vi "guardadoarchivocompleto2.vi"(0 "nombre":string, 1 "lockin":dbl[](array[numeric]), 2 "multimetro":bool, 3 "CCD":dbl[][](array[numeric]), 5 "titulo grupo":string, 6 "voltaje":dbl[](array[numeric]), 7 "potenciometro":dbl[](array[numeric]), 8 "angulo":dbl[](array[numeric]), 9 "division":dbl[](array[numeric]), 10 "Enum":T1(ring), 11 "Orden":T2(array[ring])=[enum."espejos", enum."voltaje", enum."polarizador", enum."potenciometro "], 12 "polarizador":dbl[](array[numeric]), 13 "corriente":dbl[](array[numeric]), 14 "multim.":dbl[](array[numeric]), 15 "guardar corriente":bool) -> ()   [LabVIEW 2016]
doc: "En este subVI se realiza el guardado de la información de acuerdo con el dispositivo que se encuentre en penultimo lugar y si en ultimo lugar se encuentra la CCD. \n\nLas entradas son:\nLa cadena de nombre, en la que se especifica el nombre del archivo.\nLa cadena de nombre de los grupos que se van a realizar, en caso de que la cadena llegue vacía entoces no se forman ningún grupo."
uses:
  <vilib>/UPVI/lvhdf5/file.llb/LVH5F Operation.ctl
  <vilib>/Utility/miscctls.llb/LVRectTypeDef.ctl
  <vilib>/UPVI/lvhdf5/attribute.llb/LVH5A Operation.ctl
  <vilib>/UPVI/lvhdf5/group.llb/H5G_obj_t.ctl
  <vilib>/UPVI/lvhdf5/dataset.llb/LVH5D Operation.ctl
  <vilib>/UPVI/lvhdf5/identifier.llb/Not an HDF5 Refnum Constant.vi
  <vilib>/UPVI/lvhdf5/common.llb/To HDF5 Ref.vi
  <vilib>/UPVI/lvhdf5/group.llb/OpenCreateGroup (String).vi
  <vilib>/UPVI/lvhdf5/utility.llb/Select HDF5 Dialog.vi
  <vilib>/UPVI/lvhdf5/utility.llb/Select HDF5 Dialog (Object Only).vi
  <vilib>/UPVI/lvhdf5/dataset.llb/Simple H5Dwrite (Variant).vi
  <vilib>/UPVI/lvhdf5/attribute.llb/Write Multiple Attributes.vi
  <vilib>/UPVI/lvhdf5/dataset.llb/H5Dclose.vi
  <vilib>/UPVI/lvhdf5/dataset.llb/Write Dataset with Attributes.xnode
  <vilib>/UPVI/lvhdf5/library.llb/HDF5 Ref.ctl
  <vilib>/Utility/error.llb/Error Cluster From Error Code.vi
  <vilib>/UPVI/lvhdf5/dataset.llb/OpenCreateReplace Dataset by Element Type.vi
  <vilib>/UPVI/lvhdf5/dataspace.llb/H5Sselect_hyperslab.vi
  <vilib>/UPVI/lvhdf5/dataset.llb/H5Dwrite (Variant).vi
  <vilib>/UPVI/lvhdf5/dataset.llb/H5Dget_space.vi
  <vilib>/UPVI/lvhdf5/attribute.llb/private/LVH5AwriteWDTAttrs.vi
  <vilib>/UPVI/lvhdf5/dataspace.llb/H5Sclose.vi
  <vilib>/UPVI/lvhdf5/utility.llb/Select HDF5 Dialog (File and Object).vi
  <vilib>/Utility/VariantDataType/GetClusterInfo.vi
  <vilib>/Utility/VariantDataType/VariantType.lvlib
  <vilib>/Utility/VariantDataType/GetTypeInfo.vi
  <vilib>/UPVI/lvhdf5/attribute.llb/Cluster to Attribute Array.xnode
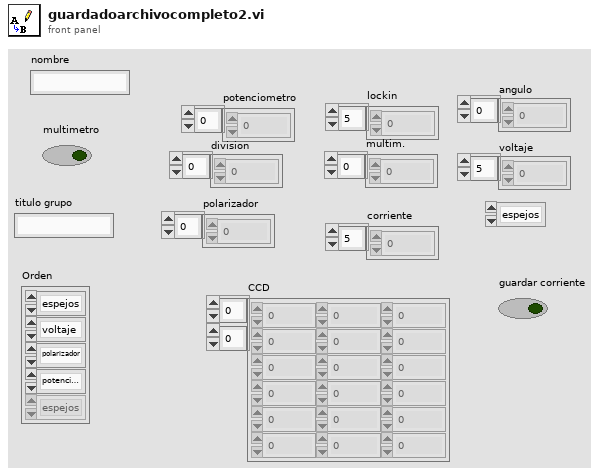
[diagram p1: front panel]
types:
  T1 = enum16{"espejos", "polarizador", "voltaje", "potenciometro ", "CCD", "lockin", "laser", "ninguno"}
  T2 = enum16{"espejos", "polarizador", "voltaje", "potenciometro ", "CCD", "lockin", "laser", "ninguno"}[]
  T3 = typedef "LVH5F Operation.ctl" = enum16{"open", "open or create", "create or replace", "create or replace (with confirmation)", "create", "open (read only)"}
  T4 = typedef "HDF5 Ref.ctl" = refnum<k1>
  T5 = typedef "LVH5A Operation.ctl" = enum16{"open", "replace", "create", "open or create", "create or replace", "create or replace with confirmation"}
  T6 = typedef "LVRectTypeDef.ctl" = cluster{"Left":i16, "Top":i16, "Right":i16, "Bottom":i16}
  T7 = cluster{"Behavior":enum32{"Invalid", "Default", "Floating", "Floating/Auto-Hide", "Modal"}, "Position":T6, "Center":bool, "Title":string}
  T8 = typedef "LVH5D Operation.ctl" = enum16{"open", "replace", "create", "open or create", "create or replace", "create or replace with confirmation"}
  T9 = typedef "H5G_obj_t.ctl" = i32
  T10 = cluster{"Object Types (any)":T9[], "Object Pattern":string}
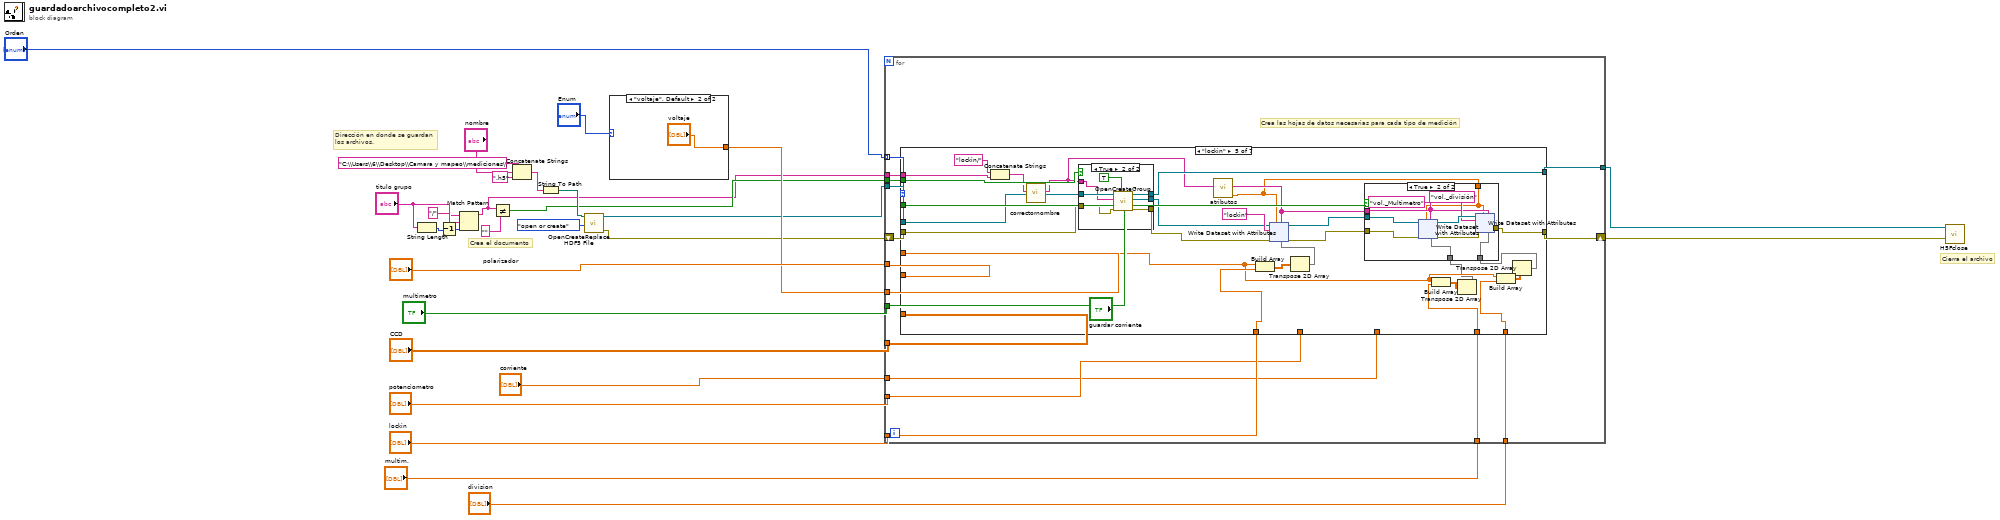
[diagram p0: block diagram]
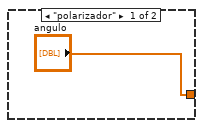
[diagram p2: hidden frame]
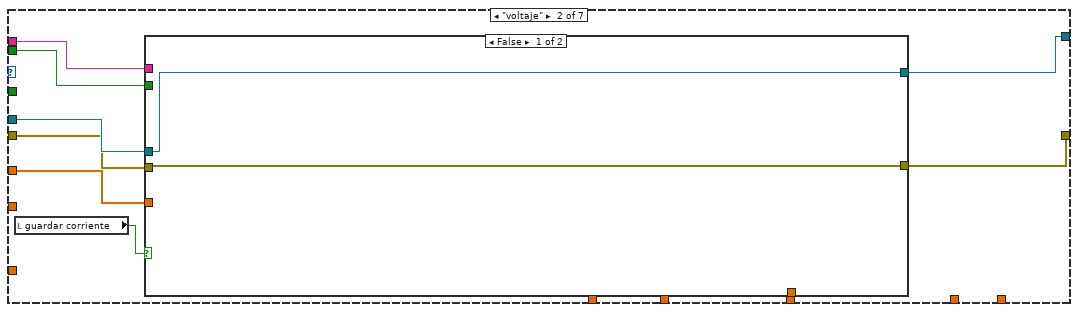
[diagram p4: hidden frame]
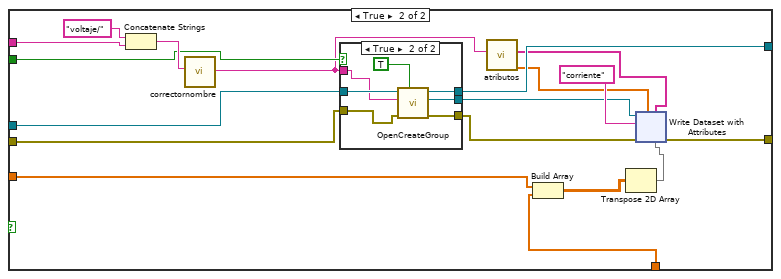
[diagram p5: hidden frame]
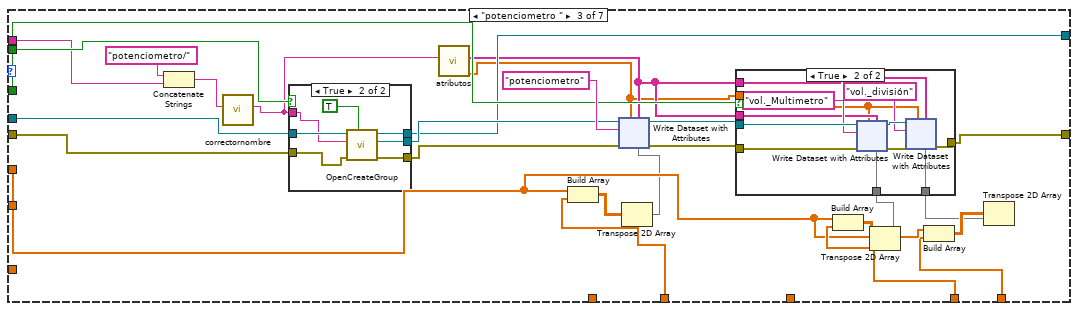
[diagram p7: hidden frame]
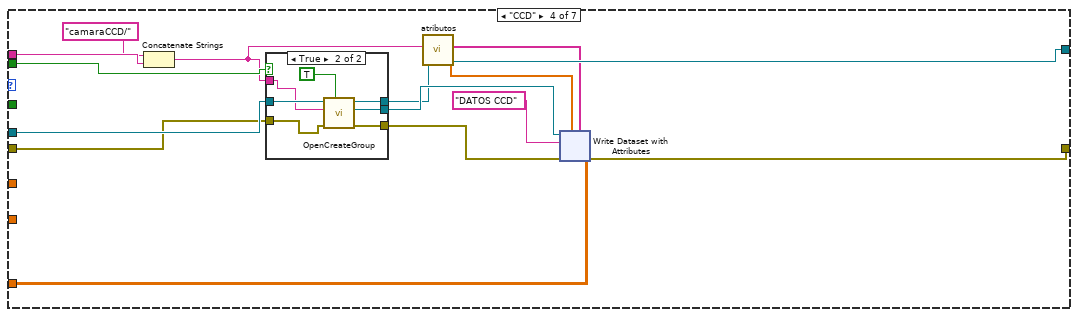
[diagram p10: hidden frame]
diagram:
  # "Dirección en donde se guardan \nlos archivos."
  # "Cierra el archivo"
  # "Crea el documento"
  n1 = String Length(string="titulo grupo") -> (length=w15:i32)
  n2 = Decrement(x=w15) -> (x-1=w16:i32)
  n3 = Match Pattern(string="titulo grupo", regular expression="/", offset (0)=w16) -> (before substring=w2:string)  [unwired: 3 out]
  n4 = Not Equal?(x=w2, y="") -> (x != y?=w3:bool)
  n5 = Concatenate Strings("C:\\Users\\6\\Desktop\\Camara y mapeo\\mediciones\\" ("string"), "nombre", ".h5" ("string")) -> (w24:string)
  n6 = String To Path(string=w24) -> (path=w23:path)
  n7 = call <vilib>:"OpenCreateReplace HDF5 File.vi"("function (open or create)"=LVH5F_Operation."open or create", "path"=w23) -> ("error out"=w4:errorcluster, "HDF5 Ref out"=w5:T4)  [unwired: 6 in]
  n8 = case shown="\"voltaje\", Default" "Enum" {
    tunnel: ["angulo" "voltaje"] -> w7
    frame "polarizador" {
    }
    frame "voltaje", Default {
    }
  }
  n9 = for {
    tunnel: "polarizador" -> [w45]
    tunnel: w5 -> [w44]
    tunnel: "Orden" -> [w43] mode=indexing
    tunnel: "lockin" -> [w41]
    tunnel: "potenciometro" -> [w40]
    tunnel: "corriente" -> [w39]
    tunnel: "multimetro" -> [w38]
    tunnel: "multim." -> [w37]
    tunnel: "CCD" -> [w36]
    shift-right: [w42] -> w21
    shift-left: w4 -> [w46]
    tunnel: "division" -> [w35]
    tunnel: w7 -> [w34]
    tunnel: w3 -> [w33]
    tunnel: w2 -> [w32]
    tunnel: [w31] -> w1
    # "Crea las hojas de datos necesarias para cada tipo de medición"
    n10 = case shown="\"lockin\"" w43 {
      tunnel: w46 -> [w48 w51 w393 w1319 w1645 w2560 w2562]
      tunnel: w45 -> [_ _ _ _ _ _ _]
      tunnel: w44 -> [w47 w52 w394 w1320 w1640 w2559 w2561]
      tunnel: [w48 w57 w404 w1325 w1652 w2560 w2562] -> w42
      tunnel: w41 -> [_ _ _ _ w1650 _ _]
      tunnel: w40 -> [_ _ w402 _ _ _ _]
      tunnel: w39 -> [_ w55 _ _ _ _ _]
      tunnel: w38 -> [_ _ w403 _ w1651 _ _]
      tunnel: w37 -> [_ _ w401 _ w1649 _ _]
      tunnel: w36 -> [_ _ _ w1323 _ _ _]
      tunnel: w35 -> [_ _ w399 _ w1648 _ _]
      tunnel: w34 -> [_ w56 w400 _ w1647 _ _]
      tunnel: w33 -> [_ w53 w397 w1315 w1642 _ _]
      tunnel: w32 -> [_ w54 w395 w1322 w1641 _ _]
      tunnel: [w47 w50 w390 w1316 w1639 w2559 w2561] -> w31
      frame "espejos", Default {
      }
      frame "voltaje" {
        n11 = local read "guardar corriente"() -> (w49:bool)
        n12 = case shown="False" w49 {
          tunnel: [w59 w76] -> w57
          tunnel: w56 -> [_ w75]
          tunnel: w55 -> [_ w74]
          tunnel: w54 -> [_ w71]
          tunnel: w53 -> [_ w70]
          tunnel: w52 -> [w58 w69]
          tunnel: w51 -> [w59 w68]
          tunnel: [w58 w65] -> w50
          frame False {
          }
          frame True {
            n13 = Concatenate Strings("voltaje/", w71) -> (w72:string)
            n14 = call "correctornombre.vi"("NUEVA"=w72) -> ("concatenated string"=w62:string)  [unwired: 10 in]
            n15 = case shown="True" w70 {
              tunnel: w69 -> [w373 w380]
              tunnel: w68 -> [w372 w379]
              tunnel: [w372 w378] -> w67
              tunnel: [w373 w377] -> w66
              tunnel: [w373 w375] -> w65
              tunnel: w62 -> [_ w374]
              frame False {
              }
              frame True {
                n16 = call-poly <vilib>:"OpenCreateGroup.vi"("Create if not found (F)"=TRUE, "error in (no error)"=w379, "Group"=w374, "HDF5 Ref"=w380) -> ("error out"=w378:errorcluster, "HDF5 Group Ref"=w377:T4, "HDF5 Ref out"=w375:T4)  [unwired: 5 in]
              }
            }
            n17 = call "atributos.vi"("titulo grupo"=w62) -> ("Array 2"=w60:dbl[], "Array"=w61:string[])  [unwired: 9 in]
            n18 = Build Array(w75, w74) -> (w63:dbl[][])
            n19 = Transpose 2D Array(2D array=w63) -> (transposed array=w64:dbl[][])
            n20 = xnode "Write Dataset with Attributes"("Dataset Path"="corriente", "error in (no error)"=w67, "HDF5 Path or Ref"=w66, "Attribute Name(s)"=w61, "Attribute Value(s)"=w60, "Data"=w64) -> ("error out"=w76:errorcluster)  [unwired: 2 in, 2 out]
          }
        }
      }
      frame "potenciometro " {
        n21 = Concatenate Strings("potenciometro/", w395) -> (w398:string)
        n22 = call "correctornombre.vi"("NUEVA"=w398) -> ("concatenated string"=w383:string)  [unwired: 10 in]
        n23 = case shown="True" w397 {
          tunnel: w394 -> [w703 w710]
          tunnel: w393 -> [w702 w709]
          tunnel: [w702 w708] -> w392
          tunnel: [w703 w707] -> w391
          tunnel: [w703 w705] -> w390
          tunnel: w383 -> [_ w704]
          frame False {
          }
          frame True {
            n24 = call-poly <vilib>:"OpenCreateGroup.vi"("Create if not found (F)"=TRUE, "error in (no error)"=w709, "Group"=w704, "HDF5 Ref"=w710) -> ("error out"=w708:errorcluster, "HDF5 Group Ref"=w707:T4, "HDF5 Ref out"=w705:T4)  [unwired: 5 in]
          }
        }
        n25 = call "atributos.vi"("titulo grupo"=w383) -> ("Array 2"=w381:dbl[], "Array"=w382:string[])  [unwired: 9 in]
        n26 = Build Array(w400, w402) -> (w389:dbl[][])
        n27 = Transpose 2D Array(2D array=w389) -> (transposed array=w388:dbl[][])
        n28 = xnode "Write Dataset with Attributes"("Dataset Path"="potenciometro", "error in (no error)"=w392, "HDF5 Path or Ref"=w391, "Attribute Name(s)"=w382, "Attribute Value(s)"=w381, "Data"=w388) -> ("HDF5 Ref out"=w406:T4, "error out"=w405:errorcluster)  [unwired: 2 in, 1 out]
        n29 = Build Array(w400, w401) -> (w387:dbl[][])
        n30 = Transpose 2D Array(2D array=w387) -> (transposed array=w386:dbl[][])
        n31 = Build Array(w400, w399) -> (w385:dbl[][])
        n32 = Transpose 2D Array(2D array=w385) -> (transposed array=w384:dbl[][])
        n33 = case shown="True" w403 {
          tunnel: w405 -> [w711 w723]
          tunnel: w406 -> [_ w722]
          tunnel: [w711 w718] -> w404
          tunnel: w386 -> [_ w716]
          tunnel: w384 -> [_ w715]
          tunnel: w382 -> [_ w714]
          tunnel: w382 -> [_ w713]
          tunnel: w381 -> [_ w712]
          frame False {
          }
          frame True {
            n34 = xnode "Write Dataset with Attributes"("Dataset Path"="vol._Multimetro", "error in (no error)"=w723, "HDF5 Path or Ref"=w722, "Attribute Name(s)"=w714, "Attribute Value(s)"=w712, "Data"=w716) -> ("HDF5 Ref out"=w719:T4, "error out"=w720:errorcluster)  [unwired: 2 in, 1 out]
            n35 = xnode "Write Dataset with Attributes"("Dataset Path"="vol._división", "error in (no error)"=w720, "HDF5 Path or Ref"=w719, "Attribute Name(s)"=w713, "Attribute Value(s)"=w712, "Data"=w715) -> ("error out"=w718:errorcluster)  [unwired: 2 in, 2 out]
          }
        }
      }
      frame "CCD" {
        n36 = Concatenate Strings("camaraCCD/" ("string"), w1322) -> (w1314:string)
        n37 = case shown="True" w1315 {
          tunnel: w1320 -> [w1621 w1628]
          tunnel: w1319 -> [w1620 w1627]
          tunnel: [w1620 w1626] -> w1318
          tunnel: [w1621 w1625] -> w1317
          tunnel: [w1621 w1623] -> w1316
          tunnel: w1314 -> [_ w1622]
          frame False {
          }
          frame True {
            n38 = call-poly <vilib>:"OpenCreateGroup.vi"("Create if not found (F)"=TRUE, "error in (no error)"=w1627, "Group"=w1622, "HDF5 Ref"=w1628) -> ("error out"=w1626:errorcluster, "HDF5 Group Ref"=w1625:T4, "HDF5 Ref out"=w1623:T4)  [unwired: 5 in]
          }
        }
        n39 = call "atributos.vi"("titulo grupo"=w1314) -> ("Array 2"=w1312:dbl[], "Array"=w1313:string[])  [unwired: 9 in]
        n40 = xnode "Write Dataset with Attributes"("Dataset Path"="DATOS CCD", "error in (no error)"=w1318, "HDF5 Path or Ref"=w1317, "Attribute Name(s)"=w1313, "Attribute Value(s)"=w1312, "Data"=w1323) -> ("error out"=w1325:errorcluster)  [unwired: 2 in, 2 out]
      }
      frame "lockin" {
        n41 = Concatenate Strings("lockin/", w1641) -> (w1638:string)
        n42 = call "correctornombre.vi"("NUEVA"=w1638) -> ("concatenated string"=w1631:string)  [unwired: 10 in]
        n43 = case shown="True" w1642 {
          tunnel: w1640 -> [w1951 w1958]
          tunnel: w1645 -> [w1950 w1957]
          tunnel: [w1950 w1956] -> w1644
          tunnel: [w1951 w1955] -> w1646
          tunnel: [w1951 w1953] -> w1639
          tunnel: w1631 -> [_ w1952]
          frame False {
          }
          frame True {
            n44 = call-poly <vilib>:"OpenCreateGroup.vi"("Create if not found (F)"=TRUE, "error in (no error)"=w1957, "Group"=w1952, "HDF5 Ref"=w1958) -> ("error out"=w1956:errorcluster, "HDF5 Group Ref"=w1955:T4, "HDF5 Ref out"=w1953:T4)  [unwired: 5 in]
          }
        }
        n45 = call "atributos.vi"("titulo grupo"=w1631) -> ("Array 2"=w1629:dbl[], "Array"=w1630:string[])  [unwired: 9 in]
        n46 = Build Array(w1647, w1650) -> (w1637:dbl[][])
        n47 = Transpose 2D Array(2D array=w1637) -> (transposed array=w1636:dbl[][])
        n48 = xnode "Write Dataset with Attributes"("Dataset Path"="lockin", "error in (no error)"=w1644, "HDF5 Path or Ref"=w1646, "Attribute Name(s)"=w1630, "Attribute Value(s)"=w1629, "Data"=w1636) -> ("HDF5 Ref out"=w1654:T4, "error out"=w1653:errorcluster)  [unwired: 2 in, 1 out]
        n49 = Build Array(w1647, w1649) -> (w1635:dbl[][])
        n50 = Transpose 2D Array(2D array=w1635) -> (transposed array=w1634:dbl[][])
        n51 = Build Array(w1647, w1648) -> (w1633:dbl[][])
        n52 = Transpose 2D Array(2D array=w1633) -> (transposed array=w1632:dbl[][])
        n53 = case shown="True" w1651 {
          tunnel: w1653 -> [w1959 w1970]
          tunnel: w1654 -> [_ w1969]
          tunnel: [w1959 w1965] -> w1652
          tunnel: w1634 -> [_ w1963]
          tunnel: w1632 -> [_ w1962]
          tunnel: w1630 -> [_ w1961]
          tunnel: w1629 -> [_ w1960]
          frame False {
          }
          frame True {
            n54 = xnode "Write Dataset with Attributes"("Dataset Path"="vol._Multimetro", "error in (no error)"=w1970, "HDF5 Path or Ref"=w1969, "Attribute Name(s)"=w1961, "Attribute Value(s)"=w1960, "Data"=w1963) -> ("HDF5 Ref out"=w1966:T4, "error out"=w1967:errorcluster)  [unwired: 2 in, 1 out]
            n55 = xnode "Write Dataset with Attributes"("Dataset Path"="vol._división", "error in (no error)"=w1967, "HDF5 Path or Ref"=w1966, "Attribute Name(s)"=w1961, "Attribute Value(s)"=w1960, "Data"=w1962) -> ("error out"=w1965:errorcluster)  [unwired: 2 in, 2 out]
          }
        }
      }
      frame "laser" {
      }
      frame "ninguno" {
      }
    }
  }
  n56 = call <vilib>:"H5Fclose.vi"("error in (no error)"=w21, "HDF5 Ref"=w1) -> ()  [unwired: 7 in, 1 out]
